vi "GetParam.vi"(8 "error in (no error)":errorcluster caption="entrée d'erreur (pas d'erreur)", 11 "AdditiveChi2Sampler.lvclass":refnum<class "AdditiveChi2Sampler.lvclass">) -> (0 "error out":errorcluster caption="sortie d'erreur", 2 "AdditiveChi2Sampler":T1={"sample_steps"=2, "sample_interval"=-1.0} {"sample_interval" min=-1.0}, 3 "AdditiveChi2Sampler.lvclass":refnum<class "AdditiveChi2Sampler.lvclass">)   [LabVIEW 2020, in "AdditiveChi2Sampler.lvclass"]
doc: "Get Parameters"
uses:
  AdditiveChi2Sampler.lvclass
  AdditiveChi2Sampler.lvclass/AdditiveChi2Sampler.ctl
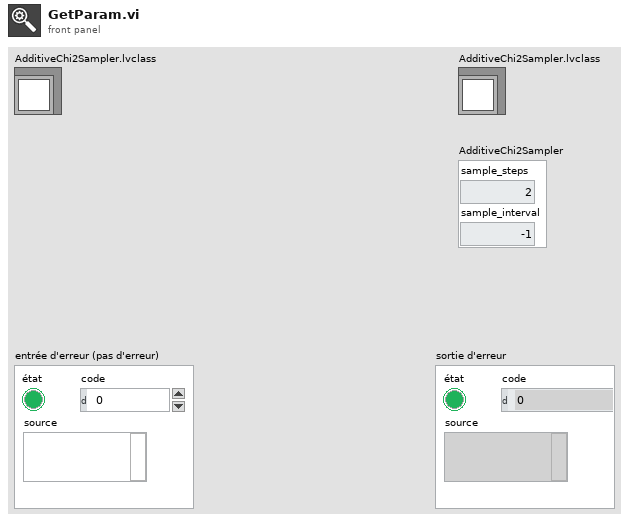
[diagram p1: front panel]
types:
  T1 = cluster{"sample_steps":i32, "sample_interval":dbl}
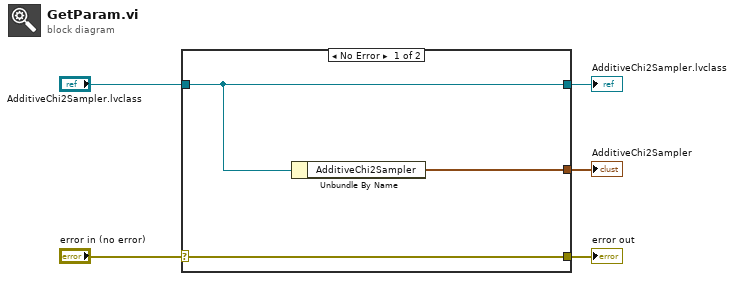
[diagram p0: block diagram]
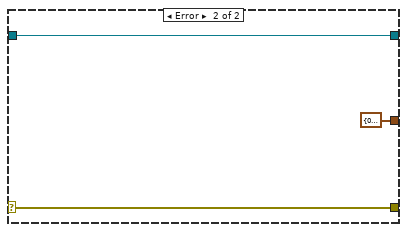
[diagram p2: hidden frame]
diagram:
  n1 = case shown="No Error" "error in (no error)" {
    selector: "error in (no error)" -> [w8 w10]
    tunnel: [w8 w10] -> w4
    tunnel: [w7 w11] -> w2
    tunnel: "AdditiveChi2Sampler.lvclass" -> [w7 w11]
    tunnel: [w6 T1 {"sample_steps"=0, "sample_interval"=0.0} ("AdditiveChi2Sampler")] -> w1
    frame No Error {
      n2 = Unbundle By Name(w7) -> ("AdditiveChi2Sampler"=w6:T1)
    }
    frame Error {
    }
  }
  "error out" <- w4
  "AdditiveChi2Sampler.lvclass" <- w2
  "AdditiveChi2Sampler" <- w1
